vi "serial_transmitter.vi"(2 "stop transmission":bool, 3 "write buffer":string) -> (0 "return count":u32, 1 "sucess":bool)   [LabVIEW 2014]
uses:
  <vilib>/Instr/_visa.llb/VISA Open Access Mode.ctl
panel:
  in  "Access Mode":T1 items=["VISA Defaults"=0, "Exclusive Lock"=1, "Load Configured Settings"=4]
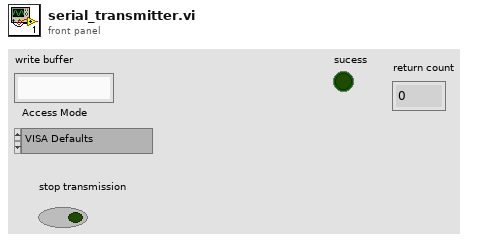
[diagram p1: front panel]
types:
  T1 = typedef "VISA Open Access Mode.ctl" = u32
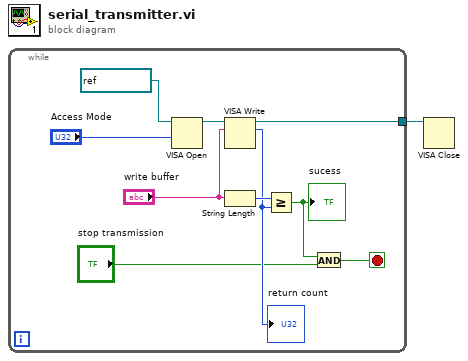
[diagram p0: block diagram]
diagram:
  n1 = while {
    tunnel: [w2] -> w1
    stop <- w3 stop-if-true
    n2 = VISA Open(access mode="Access Mode", VISA resource name=refnum<visa-resource-name> "COM1") -> (VISA resource name=w10:refnum<visa-resource-name>)  [unwired: 3 in, 1 out]
    n3 = VISA Write(VISA resource name=w10, write buffer="write buffer") -> (VISA resource name out=w2:refnum<visa-resource-name>, return count=w6:u32)  [unwired: 1 in, 1 out]
    "return count" <- w6
    n4 = String Length(string="write buffer") -> (length=w7:i32)
    n5 = Greater Or Equal?(x=w7, y=w6) -> (x >= y?=w5:bool)
    "sucess" <- w5
    n6 = And(x=w5, y="stop transmission") -> (x .and. y?=w3:bool)
  }
  n7 = VISA Close(VISA resource name=w1) -> ()  [unwired: 1 in, 1 out]
